vi "MI Cryostation 1.4 LV v14.vi"(6 "Temperature Set Point":dbl[unit]=4.2 min=2.0 max=350.0 step=1.0 format="%.2f", 9 "Address":string="localhost") -> (0 "Platform Stability":dbl[unit]=-0.1 format="%1.2f", 1 "Platform":dbl[unit]=-0.1 format="%1.3f", 2 "Sample Stability":dbl[unit]=-0.1 format="%1.2f", 3 "Sample":dbl[unit]=-0.1 format="%1.3f", 5 "Set Point":dbl[unit]=-0.1 format="%1.2f")   [LabVIEW 2014]
doc: "Displays data sent via TCP from Data Server.vi. Once a TCP connection is open, the VI reads 4 bytes to determine the amount of data being sent. It then reads and charts that many bytes. If an error occurs or the stop button is pressed, it sends a \"Q\" to the Data Sender to notify it to quit.\n\n<B>Note:</B> Requires the Data Server.vi located in the same library as this VI."
panel:
  out "Alarm":bool
  in  "Set Magnet Target Field":bool caption="Send"
  in  "Magnet Target Field":dbl[unit] min=-2.0 max=2.0 format="%.3f"
  in  "Magnet Disable":bool
  in  "Magnet Enable":bool
  out "Magnet Target Field":dbl[unit]=-9.999999 format="%1.3f"
  out "Magnet State":string="Unknown"
  out "Magnet":string="Magnet"
  in  "Standby":bool
  out "Heater Power":dbl[unit]=-0.1 format="%1.3f"
  out "User":dbl[unit]=-0.1 format="%1.3f"
  out "User Stability":dbl[unit]=-0.1 format="%1.2f"
  in  "Set Temperature Set Point":bool
  in  "stop":bool
  in  "Stop":bool
  in  "WarmUp":bool
  in  "CoolDown":bool
  out "Stability":string="Stability"
  out "Temperature":string="Temperature"
  out "Temperature Graph":cluster{dbl[unit], dbl[unit], dbl[unit]}(graph)
  # "Input the IP address of the Cryostation PC"
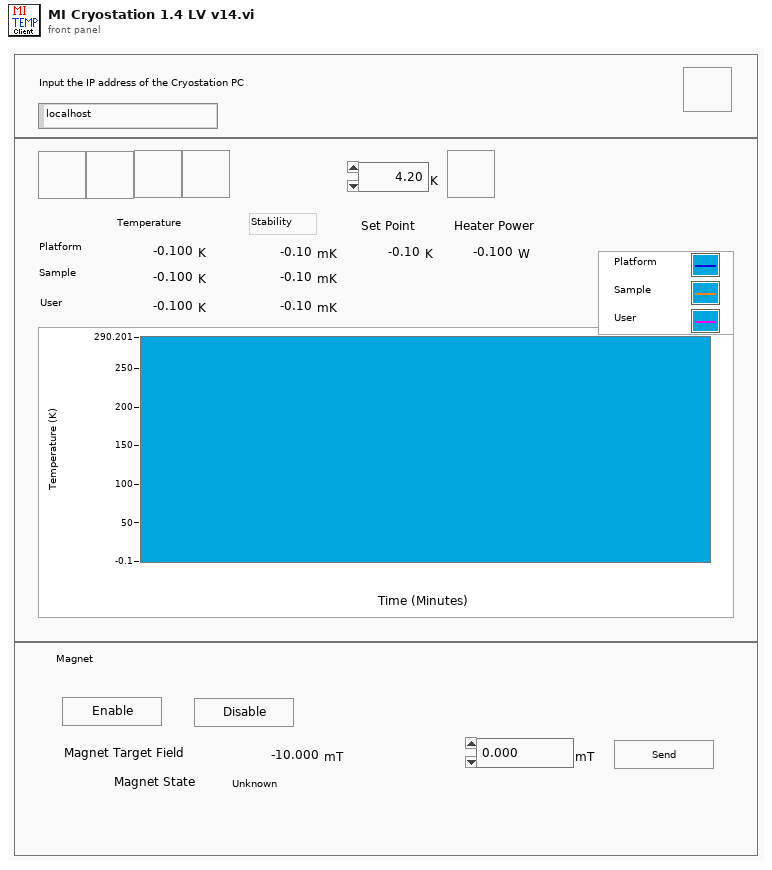
[diagram p1: front panel]
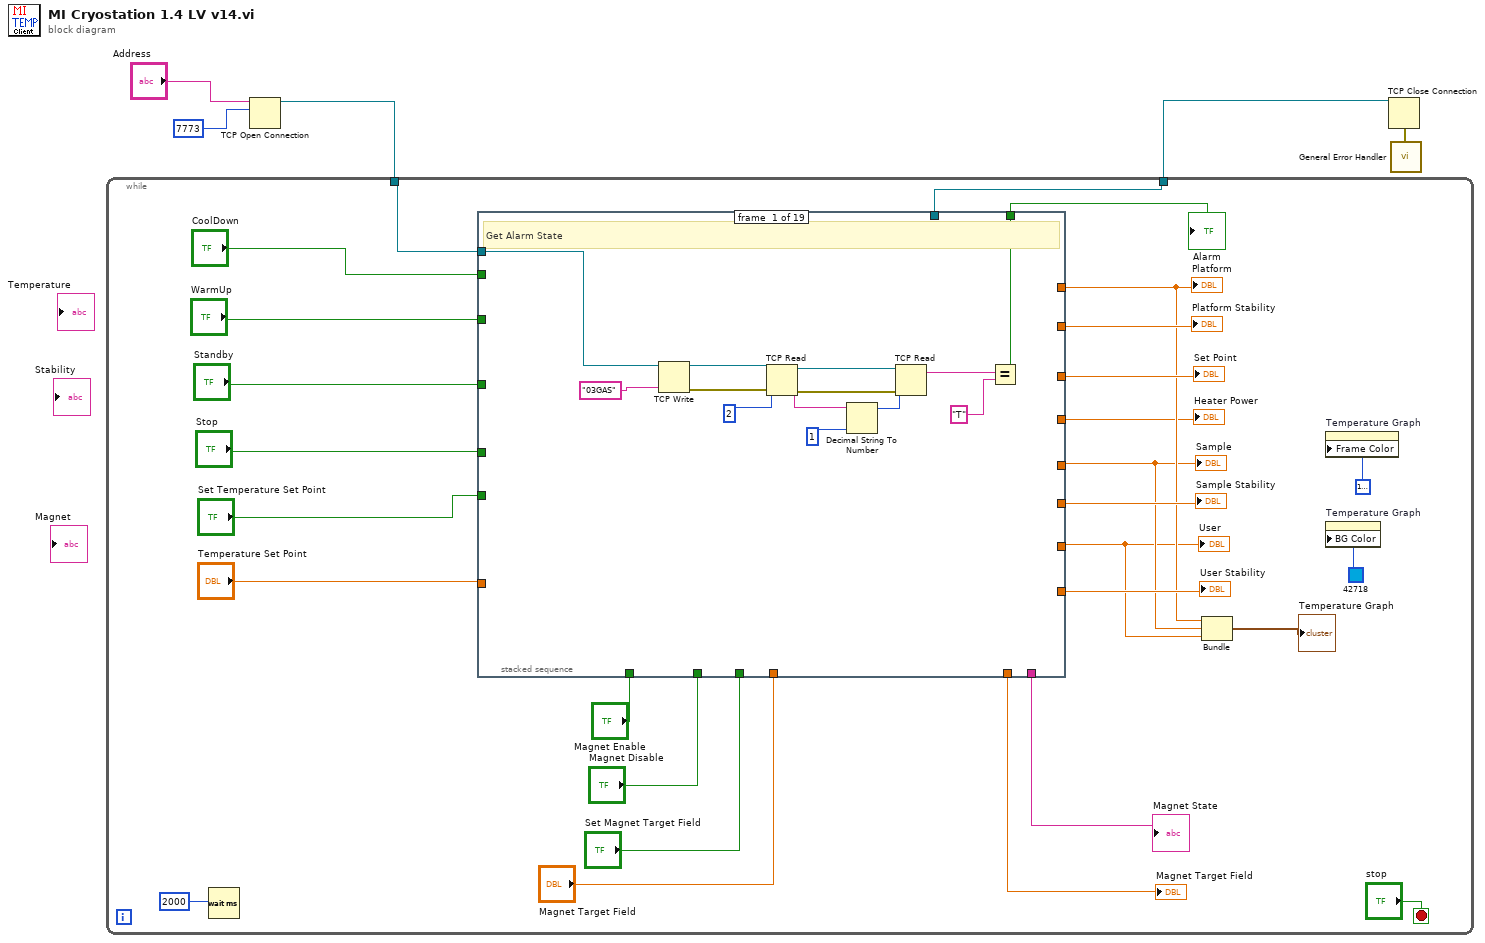
[diagram p0: block diagram]
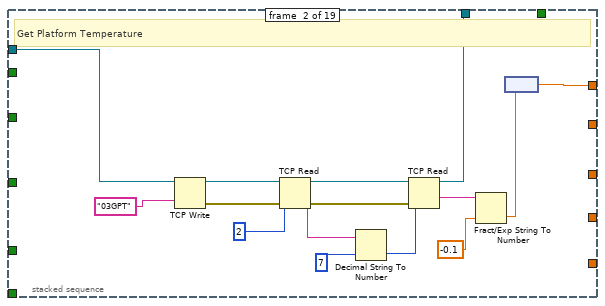
[diagram p2: hidden frame]
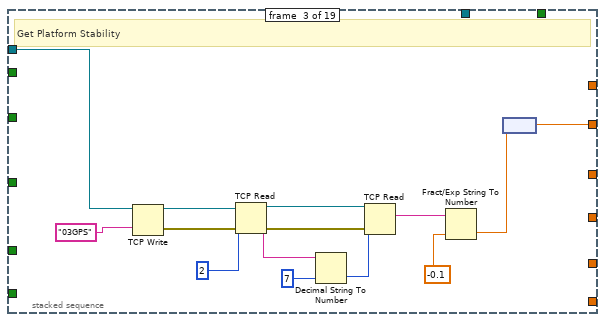
[diagram p3: hidden frame]
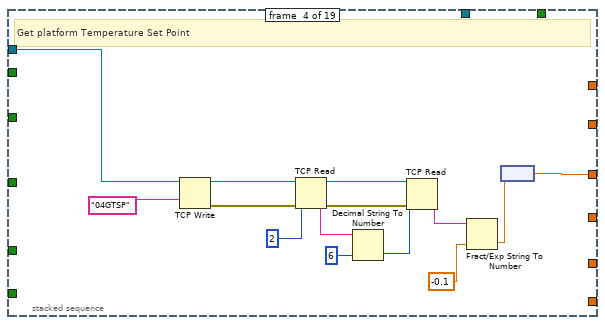
[diagram p4: hidden frame]
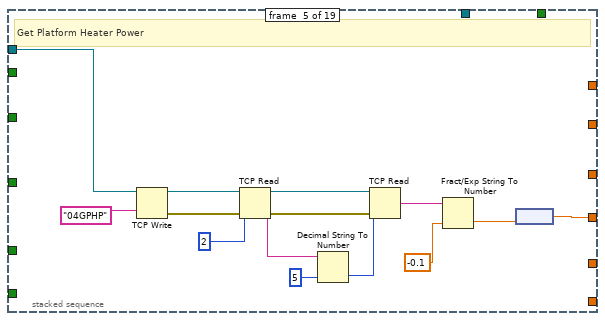
[diagram p5: hidden frame]
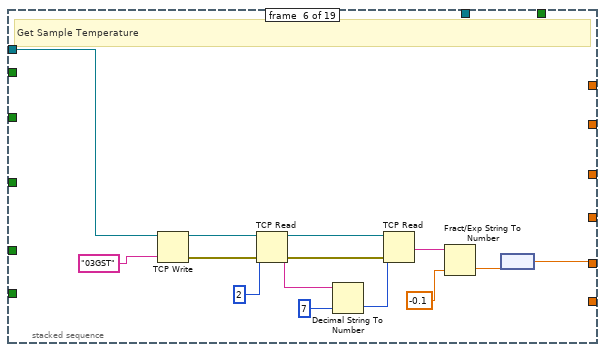
[diagram p6: hidden frame]
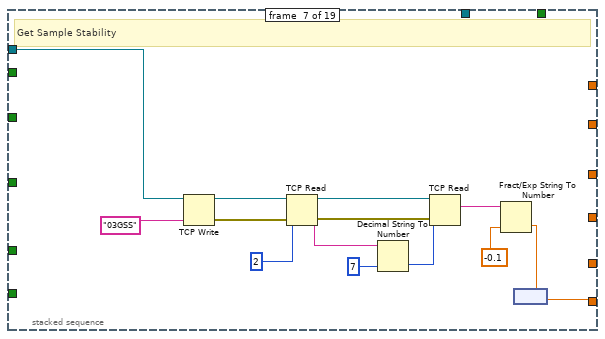
[diagram p7: hidden frame]
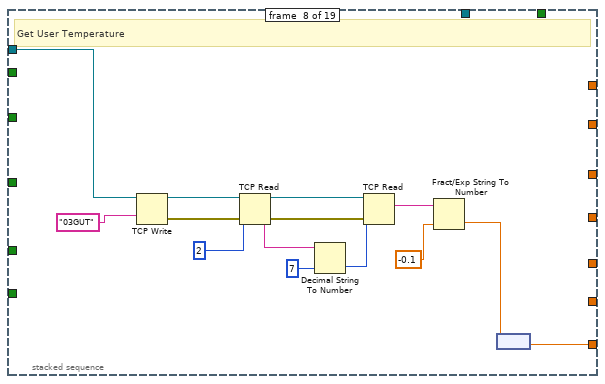
[diagram p8: hidden frame]
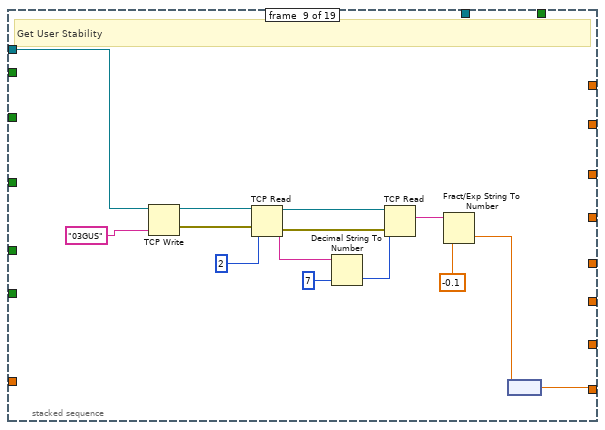
[diagram p9: hidden frame]
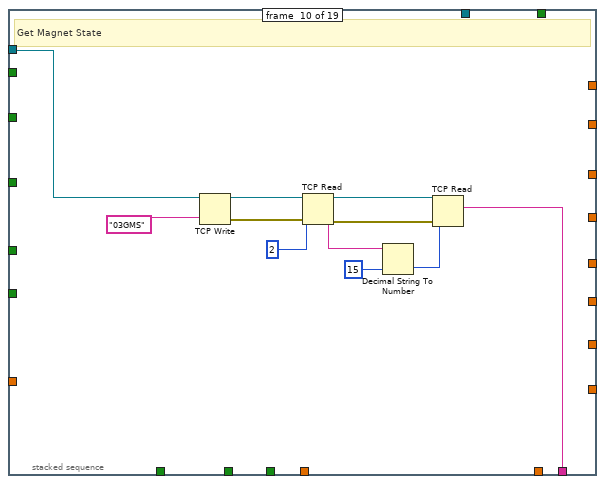
[diagram p10: hidden frame]
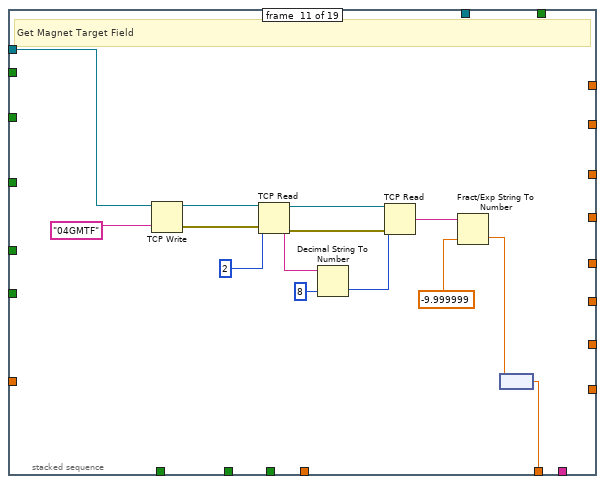
[diagram p11: hidden frame]
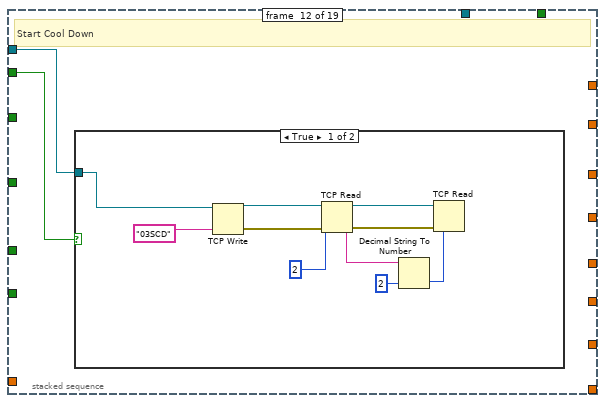
[diagram p12: hidden frame]
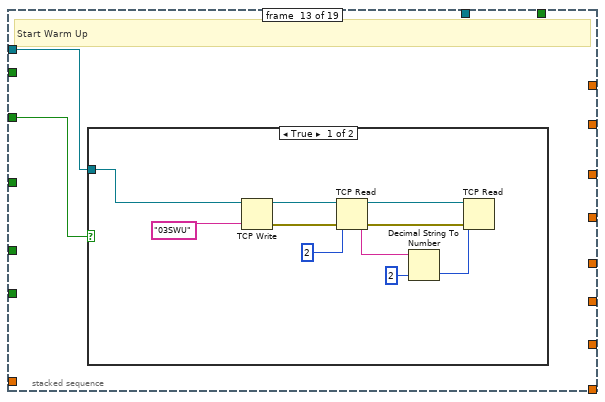
[diagram p14: hidden frame]
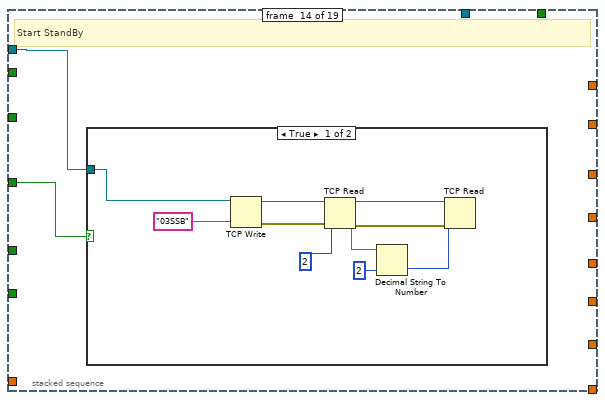
[diagram p16: hidden frame]
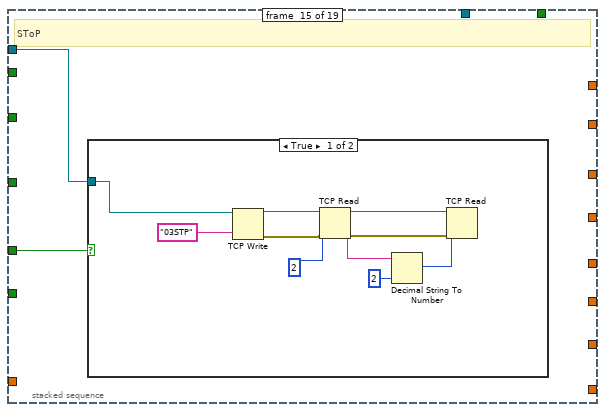
[diagram p18: hidden frame]
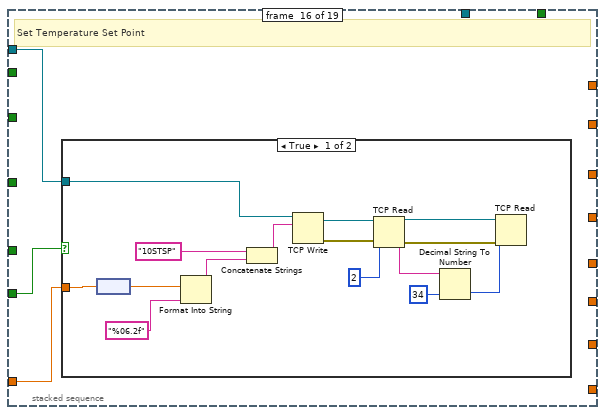
[diagram p20: hidden frame]
diagram:
  n1 = TCP Open Connection(address="Address", remote port or service name=u16 7773) -> (connection ID=w4:refnum<k5>)  [unwired: 3 in, 1 out]
  n2 = while {
    tunnel: w4 -> [w33]
    tunnel: [w30] -> w3
    stop <- "stop" stop-if-true
    n3 = Wait (ms)(milliseconds to wait=u32 2000) -> ()  [unwired: 1 out]
    n4 = stacked-sequence {
      tunnel: w33 -> [w45 w58 w72 w86 w100 w116 w128 w142 w156 w164 w177 w185 w197 w209 w221 w235 w252 w264 w277]
      tunnel: [_ _ _ w80 _ _ _ _ _ _ _ _ _ _ _ _ _ _ _] -> w26
      tunnel: "Set Temperature Set Point" -> [_ _ _ _ _ _ _ _ _ _ _ _ _ _ _ w234 _ _ _]
      tunnel: "Temperature Set Point" -> [_ _ _ _ _ _ _ _ _ _ _ _ _ _ _ w233 _ _ _]
      tunnel: [_ _ _ _ _ _ w122 _ _ _ _ _ _ _ _ _ _ _ _] -> w32
      tunnel: [_ w51 _ _ _ _ _ _ _ _ _ _ _ _ _ _ _ _ _] -> w21
      tunnel: [_ _ w67 _ _ _ _ _ _ _ _ _ _ _ _ _ _ _ _] -> w31
      tunnel: [_ _ _ _ _ w108 _ _ _ _ _ _ _ _ _ _ _ _ _] -> w20
      tunnel: [_ w53 _ _ _ _ _ _ _ _ _ _ _ _ _ _ _ _ _] -> w30
      tunnel: [_ _ _ _ _ _ _ w136 _ _ _ _ _ _ _ _ _ _ _] -> w19
      tunnel: [_ _ _ _ _ _ _ _ w150 _ _ _ _ _ _ _ _ _ _] -> w24
      tunnel: [_ _ _ _ w95 _ _ _ _ _ _ _ _ _ _ _ _ _ _] -> w6
      tunnel: "CoolDown" -> [_ _ _ _ _ _ _ _ _ _ _ w186 _ _ _ _ _ _ _]
      tunnel: "WarmUp" -> [_ _ _ _ _ _ _ _ _ _ _ _ w198 _ _ _ _ _ _]
      tunnel: "Standby" -> [_ _ _ _ _ _ _ _ _ _ _ _ _ w210 _ _ _ _ _]
      tunnel: "Stop" -> [_ _ _ _ _ _ _ _ _ _ _ _ _ _ w222 _ _ _ _]
      tunnel: [_ _ _ _ _ _ _ _ _ w163 _ _ _ _ _ _ _ _ _] -> w16
      tunnel: [_ _ _ _ _ _ _ _ _ _ w175 _ _ _ _ _ _ _ _] -> w15
      tunnel: "Magnet Enable" -> [_ _ _ _ _ _ _ _ _ _ _ _ _ _ _ _ w251 _ _]
      tunnel: "Magnet Disable" -> [_ _ _ _ _ _ _ _ _ _ _ _ _ _ _ _ _ w263 _]
      tunnel: "Set Magnet Target Field" -> [_ _ _ _ _ _ _ _ _ _ _ _ _ _ _ _ _ _ w275]
      tunnel: "Magnet Target Field" -> [_ _ _ _ _ _ _ _ _ _ _ _ _ _ _ _ _ _ w276]
      tunnel: [w40 _ _ _ _ _ _ _ _ _ _ _ _ _ _ _ _ _ _] -> w11
      frame #0 {
        # "Get Alarm State"
        n5 = TCP Write(connection ID=w45, data in="03GAS") -> (connection ID out=w39:refnum<k5>, error out=w38:errorcluster)  [unwired: 2 in, 1 out]
        n6 = TCP Read(connection ID=w39, bytes to read=2, error in (no error)=w38) -> (connection ID out=w43:refnum<k5>, data out=w34:string, error out=w37:errorcluster)  [unwired: 2 in]
        n7 = Decimal String To Number(string=w34, default (0L)=1 ("default (0 I32)")) -> (number=w35:i32)  [unwired: 1 in, 1 out]
        n8 = TCP Read(connection ID=w43, bytes to read=w35, error in (no error)=w37) -> (data out=w42:string)  [unwired: 2 in, 2 out]
        n9 = Equal?(x=w42, y="T") -> (x = y?=w40:bool)
      }
      frame #1 {
        # "Get Platform Temperature"
        n10 = TCP Write(connection ID=w58, data in="03GPT") -> (connection ID out=w61:refnum<k5>, error out=w50:errorcluster)  [unwired: 2 in, 1 out]
        n11 = TCP Read(connection ID=w61, bytes to read=2, error in (no error)=w50) -> (connection ID out=w56:refnum<k5>, data out=w57:string, error out=w49:errorcluster)  [unwired: 2 in]
        n12 = Decimal String To Number(string=w57, default (0L)=7 ("default (0 I32)")) -> (number=w55:i32)  [unwired: 1 in, 1 out]
        n13 = TCP Read(connection ID=w56, bytes to read=w55, error in (no error)=w49) -> (connection ID out=w53:refnum<k5>, data out=w54:string)  [unwired: 2 in, 1 out]
        n14 = Fract/Exp String To Number(string=w54, default (0 dbl)=-0.1 ("default (0 DBL)")) -> (number=w52:dbl)  [unwired: 2 in, 1 out]
        n15 = node(w52) -> (w51:dbl[unit])
      }
      frame #2 {
        # "Get Platform Stability"
        n16 = TCP Write(connection ID=w72, data in="03GPS") -> (connection ID out=w73:refnum<k5>, error out=w64:errorcluster)  [unwired: 2 in, 1 out]
        n17 = TCP Read(connection ID=w73, bytes to read=2, error in (no error)=w64) -> (connection ID out=w68:refnum<k5>, data out=w70:string, error out=w65:errorcluster)  [unwired: 2 in]
        n18 = Decimal String To Number(string=w70, default (0L)=7 ("default (0 I32)")) -> (number=w71:i32)  [unwired: 1 in, 1 out]
        n19 = TCP Read(connection ID=w68, bytes to read=w71, error in (no error)=w65) -> (data out=w69:string)  [unwired: 2 in, 2 out]
        n20 = Fract/Exp String To Number(string=w69, default (0 dbl)=-0.1 ("default (0 DBL)")) -> (number=w66:dbl)  [unwired: 2 in, 1 out]
        n21 = node(w66) -> (w67:dbl[unit])
      }
      frame #3 {
        # "Get platform Temperature Set Point"
        n22 = TCP Write(connection ID=w86, data in="04GTSP") -> (connection ID out=w87:refnum<k5>, error out=w79:errorcluster)  [unwired: 2 in, 1 out]
        n23 = TCP Read(connection ID=w87, bytes to read=2, error in (no error)=w79) -> (connection ID out=w84:refnum<k5>, data out=w85:string, error out=w78:errorcluster)  [unwired: 2 in]
        n24 = Decimal String To Number(string=w85, default (0L)=6 ("default (0 I32)")) -> (number=w83:i32)  [unwired: 1 in, 1 out]
        n25 = TCP Read(connection ID=w84, bytes to read=w83, error in (no error)=w78) -> (data out=w82:string)  [unwired: 2 in, 2 out]
        n26 = Fract/Exp String To Number(string=w82, default (0 dbl)=-0.1 ("default (0 DBL)")) -> (number=w81:dbl)  [unwired: 2 in, 1 out]
        n27 = node(w81) -> (w80:dbl[unit])
      }
      frame #4 {
        # "Get Platform Heater Power"
        n28 = TCP Write(connection ID=w100, data in="04GPHP") -> (connection ID out=w101:refnum<k5>, error out=w93:errorcluster)  [unwired: 2 in, 1 out]
        n29 = TCP Read(connection ID=w101, bytes to read=2, error in (no error)=w93) -> (connection ID out=w98:refnum<k5>, data out=w99:string, error out=w92:errorcluster)  [unwired: 2 in]
        n30 = Decimal String To Number(string=w99, default (0L)=5 ("default (0 I32)")) -> (number=w97:i32)  [unwired: 1 in, 1 out]
        n31 = TCP Read(connection ID=w98, bytes to read=w97, error in (no error)=w92) -> (data out=w96:string)  [unwired: 2 in, 2 out]
        n32 = Fract/Exp String To Number(string=w96, default (0 dbl)=-0.1 ("default (0 DBL)")) -> (number=w94:dbl)  [unwired: 2 in, 1 out]
        n33 = node(w94) -> (w95:dbl[unit])
      }
      frame #5 {
        # "Get Sample Temperature"
        n34 = TCP Write(connection ID=w116, data in="03GST") -> (connection ID out=w114:refnum<k5>, error out=w107:errorcluster)  [unwired: 2 in, 1 out]
        n35 = TCP Read(connection ID=w114, bytes to read=2, error in (no error)=w107) -> (connection ID out=w112:refnum<k5>, data out=w113:string, error out=w106:errorcluster)  [unwired: 2 in]
        n36 = Decimal String To Number(string=w113, default (0L)=7 ("default (0 I32)")) -> (number=w111:i32)  [unwired: 1 in, 1 out]
        n37 = TCP Read(connection ID=w112, bytes to read=w111, error in (no error)=w106) -> (data out=w110:string)  [unwired: 2 in, 2 out]
        n38 = Fract/Exp String To Number(string=w110, default (0 dbl)=-0.1 ("default (0 DBL)")) -> (number=w109:dbl)  [unwired: 2 in, 1 out]
        n39 = node(w109) -> (w108:dbl[unit])
      }
      frame #6 {
        # "Get Sample Stability"
        n40 = TCP Write(connection ID=w128, data in="03GSS") -> (connection ID out=w131:refnum<k5>, error out=w121:errorcluster)  [unwired: 2 in, 1 out]
        n41 = TCP Read(connection ID=w131, bytes to read=2, error in (no error)=w121) -> (connection ID out=w126:refnum<k5>, data out=w127:string, error out=w120:errorcluster)  [unwired: 2 in]
        n42 = Decimal String To Number(string=w127, default (0L)=7 ("default (0 I32)")) -> (number=w125:i32)  [unwired: 1 in, 1 out]
        n43 = TCP Read(connection ID=w126, bytes to read=w125, error in (no error)=w120) -> (data out=w124:string)  [unwired: 2 in, 2 out]
        n44 = Fract/Exp String To Number(string=w124, default (0 dbl)=-0.1 ("default (0 DBL)")) -> (number=w123:dbl)  [unwired: 2 in, 1 out]
        n45 = node(w123) -> (w122:dbl[unit])
      }
      frame #7 {
        # "Get User Temperature"
        n46 = TCP Write(connection ID=w142, data in="03GUT") -> (connection ID out=w145:refnum<k5>, error out=w135:errorcluster)  [unwired: 2 in, 1 out]
        n47 = TCP Read(connection ID=w145, bytes to read=2, error in (no error)=w135) -> (connection ID out=w140:refnum<k5>, data out=w141:string, error out=w134:errorcluster)  [unwired: 2 in]
        n48 = Decimal String To Number(string=w141, default (0L)=7 ("default (0 I32)")) -> (number=w139:i32)  [unwired: 1 in, 1 out]
        n49 = TCP Read(connection ID=w140, bytes to read=w139, error in (no error)=w134) -> (data out=w138:string)  [unwired: 2 in, 2 out]
        n50 = Fract/Exp String To Number(string=w138, default (0 dbl)=-0.1 ("default (0 DBL)")) -> (number=w137:dbl)  [unwired: 2 in, 1 out]
        n51 = node(w137) -> (w136:dbl[unit])
      }
      frame #8 {
        # "Get User Stability"
        n52 = TCP Write(connection ID=w156, data in="03GUS") -> (connection ID out=w159:refnum<k5>, error out=w149:errorcluster)  [unwired: 2 in, 1 out]
        n53 = TCP Read(connection ID=w159, bytes to read=2, error in (no error)=w149) -> (connection ID out=w154:refnum<k5>, data out=w155:string, error out=w148:errorcluster)  [unwired: 2 in]
        n54 = Decimal String To Number(string=w155, default (0L)=7 ("default (0 I32)")) -> (number=w153:i32)  [unwired: 1 in, 1 out]
        n55 = TCP Read(connection ID=w154, bytes to read=w153, error in (no error)=w148) -> (data out=w152:string)  [unwired: 2 in, 2 out]
        n56 = Fract/Exp String To Number(string=w152, default (0 dbl)=-0.1 ("default (0 DBL)")) -> (number=w151:dbl)  [unwired: 2 in, 1 out]
        n57 = node(w151) -> (w150:dbl[unit])
      }
      frame #9 {
        # "Get Magnet State"
        n58 = TCP Write(connection ID=w164, data in="03GMS") -> (connection ID out=w170:refnum<k5>, error out=w162:errorcluster)  [unwired: 2 in, 1 out]
        n59 = TCP Read(connection ID=w170, bytes to read=2, error in (no error)=w162) -> (connection ID out=w166:refnum<k5>, data out=w167:string, error out=w161:errorcluster)  [unwired: 2 in]
        n60 = Decimal String To Number(string=w167, default (0L)=15 ("default (0 I32)")) -> (number=w165:i32)  [unwired: 1 in, 1 out]
        n61 = TCP Read(connection ID=w166, bytes to read=w165, error in (no error)=w161) -> (data out=w163:string)  [unwired: 2 in, 2 out]
      }
      frame #10 {
        # "Get Magnet Target Field"
        n62 = TCP Write(connection ID=w177, data in="04GMTF") -> (connection ID out=w179:refnum<k5>, error out=w174:errorcluster)  [unwired: 2 in, 1 out]
        n63 = TCP Read(connection ID=w179, bytes to read=2, error in (no error)=w174) -> (connection ID out=w183:refnum<k5>, data out=w182:string, error out=w173:errorcluster)  [unwired: 2 in]
        n64 = Decimal String To Number(string=w182, default (0L)=8 ("default (0 I32)")) -> (number=w184:i32)  [unwired: 1 in, 1 out]
        n65 = TCP Read(connection ID=w183, bytes to read=w184, error in (no error)=w173) -> (data out=w178:string)  [unwired: 2 in, 2 out]
        n66 = Fract/Exp String To Number(string=w178, default (0 dbl)=-9.999999 ("default (0 DBL)")) -> (number=w176:dbl)  [unwired: 2 in, 1 out]
        n67 = node(w176) -> (w175:dbl[unit])
      }
      frame #11 {
        # "Start Cool Down"
        n68 = case shown="True" w186 {
          tunnel: w185 -> [w196 _]
          frame True {
            n69 = TCP Write(connection ID=w196, data in="03SCD") -> (connection ID out=w195:refnum<k5>, error out=w189:errorcluster)  [unwired: 2 in, 1 out]
            n70 = TCP Read(connection ID=w195, bytes to read=2 ("timeout ms (25000)"), error in (no error)=w189) -> (connection ID out=w190:refnum<k5>, data out=w192:string, error out=w188:errorcluster)  [unwired: 2 in]
            n71 = Decimal String To Number(string=w192, default (0L)=2 ("default (0 I32)")) -> (number=w191:i32)  [unwired: 1 in, 1 out]
            n72 = TCP Read(connection ID=w190, bytes to read=w191, error in (no error)=w188) -> ()  [unwired: 2 in, 3 out]
          }
          frame False {
          }
        }
      }
      frame #12 {
        # "Start Warm Up"
        n73 = case shown="True" w198 {
          tunnel: w197 -> [w208 _]
          frame True {
            n74 = TCP Write(connection ID=w208, data in="03SWU") -> (connection ID out=w207:refnum<k5>, error out=w201:errorcluster)  [unwired: 2 in, 1 out]
            n75 = TCP Read(connection ID=w207, bytes to read=2 ("timeout ms (25000)"), error in (no error)=w201) -> (connection ID out=w203:refnum<k5>, data out=w202:string, error out=w200:errorcluster)  [unwired: 2 in]
            n76 = Decimal String To Number(string=w202, default (0L)=2 ("default (0 I32)")) -> (number=w204:i32)  [unwired: 1 in, 1 out]
            n77 = TCP Read(connection ID=w203, bytes to read=w204, error in (no error)=w200) -> ()  [unwired: 2 in, 3 out]
          }
          frame False {
          }
        }
      }
      frame #13 {
        # "Start StandBy"
        n78 = case shown="True" w210 {
          tunnel: w209 -> [w220 _]
          frame True {
            n79 = TCP Write(connection ID=w220, data in="03SSB") -> (connection ID out=w219:refnum<k5>, error out=w213:errorcluster)  [unwired: 2 in, 1 out]
            n80 = TCP Read(connection ID=w219, bytes to read=2 ("timeout ms (25000)"), error in (no error)=w213) -> (connection ID out=w214:refnum<k5>, data out=w215:string, error out=w212:errorcluster)  [unwired: 2 in]
            n81 = Decimal String To Number(string=w215, default (0L)=2 ("default (0 I32)")) -> (number=w216:i32)  [unwired: 1 in, 1 out]
            n82 = TCP Read(connection ID=w214, bytes to read=w216, error in (no error)=w212) -> ()  [unwired: 2 in, 3 out]
          }
          frame False {
          }
        }
      }
      frame #14 {
        # "SToP"
        n83 = case shown="True" w222 {
          tunnel: w221 -> [w232 _]
          frame True {
            n84 = TCP Write(connection ID=w232, data in="03STP") -> (connection ID out=w231:refnum<k5>, error out=w225:errorcluster)  [unwired: 2 in, 1 out]
            n85 = TCP Read(connection ID=w231, bytes to read=2 ("timeout ms (25000)"), error in (no error)=w225) -> (connection ID out=w226:refnum<k5>, data out=w227:string, error out=w224:errorcluster)  [unwired: 2 in]
            n86 = Decimal String To Number(string=w227, default (0L)=2 ("default (0 I32)")) -> (number=w228:i32)  [unwired: 1 in, 1 out]
            n87 = TCP Read(connection ID=w226, bytes to read=w228, error in (no error)=w224) -> ()  [unwired: 2 in, 3 out]
          }
          frame False {
          }
        }
      }
      frame #15 {
        # "Set Temperature Set Point"
        n88 = case shown="True" w234 {
          tunnel: w233 -> [w240 _]
          tunnel: w235 -> [w246 _]
          frame True {
            n89 = node(w240) -> (w239:dbl)
            n90 = Format Into String(format string="%06.2f", w239) -> (resulting string=w248:string)  [unwired: 2 in, 1 out]
            n91 = Concatenate Strings("10STSP", w248) -> (w247:string)
            n92 = TCP Write(connection ID=w246, data in=w247) -> (connection ID out=w245:refnum<k5>, error out=w238:errorcluster)  [unwired: 2 in, 1 out]
            n93 = TCP Read(connection ID=w245, bytes to read=2 ("timeout ms (25000)"), error in (no error)=w238) -> (connection ID out=w243:refnum<k5>, data out=w242:string, error out=w237:errorcluster)  [unwired: 2 in]
            n94 = Decimal String To Number(string=w242, default (0L)=34 ("default (0 I32)")) -> (number=w241:i32)  [unwired: 1 in, 1 out]
            n95 = TCP Read(connection ID=w243, bytes to read=w241, error in (no error)=w237) -> ()  [unwired: 2 in, 3 out]
          }
          frame False {
          }
        }
      }
      frame #16 {
        # "Set Magnet Enabled"
        n96 = case shown="True" w251 {
          tunnel: w252 -> [w262 _]
          frame True {
            n97 = TCP Write(connection ID=w262, data in="03SME") -> (connection ID out=w261:refnum<k5>, error out=w255:errorcluster)  [unwired: 2 in, 1 out]
            n98 = TCP Read(connection ID=w261, bytes to read=2 ("timeout ms (25000)"), error in (no error)=w255) -> (connection ID out=w256:refnum<k5>, data out=w257:string, error out=w254:errorcluster)  [unwired: 2 in]
            n99 = Decimal String To Number(string=w257, default (0L)=18 ("default (0 I32)")) -> (number=w258:i32)  [unwired: 1 in, 1 out]
            n100 = TCP Read(connection ID=w256, bytes to read=w258, error in (no error)=w254) -> ()  [unwired: 2 in, 3 out]
          }
          frame False {
          }
        }
      }
      frame #17 {
        # "Set Magnet Disabled"
        n101 = case shown="True" w263 {
          tunnel: w264 -> [w274 _]
          frame True {
            n102 = TCP Write(connection ID=w274, data in="03SMD") -> (connection ID out=w273:refnum<k5>, error out=w267:errorcluster)  [unwired: 2 in, 1 out]
            n103 = TCP Read(connection ID=w273, bytes to read=2 ("timeout ms (25000)"), error in (no error)=w267) -> (connection ID out=w268:refnum<k5>, data out=w269:string, error out=w266:errorcluster)  [unwired: 2 in]
            n104 = Decimal String To Number(string=w269, default (0L)=19 ("default (0 I32)")) -> (number=w270:i32)  [unwired: 1 in, 1 out]
            n105 = TCP Read(connection ID=w268, bytes to read=w270, error in (no error)=w266) -> ()  [unwired: 2 in, 3 out]
          }
          frame False {
          }
        }
      }
      frame #18 {
        # "Set Magnet Target Field"
        n106 = case shown="True" w275 {
          tunnel: w276 -> [w282 _]
          tunnel: w277 -> [w288 _]
          frame True {
            n107 = node(w282) -> (w281:dbl)
            n108 = Format Into String(format string="%+08.6f", w281) -> (resulting string=w290:string)  [unwired: 2 in, 1 out]
            n109 = Concatenate Strings("13SMTF", w290) -> (w289:string)
            n110 = TCP Write(connection ID=w288, data in=w289) -> (connection ID out=w287:refnum<k5>, error out=w280:errorcluster)  [unwired: 2 in, 1 out]
            n111 = TCP Read(connection ID=w287, bytes to read=2 ("timeout ms (25000)"), error in (no error)=w280) -> (connection ID out=w285:refnum<k5>, data out=w284:string, error out=w279:errorcluster)  [unwired: 2 in]
            n112 = Decimal String To Number(string=w284, default (0L)=34 ("default (0 I32)")) -> (number=w283:i32)  [unwired: 1 in, 1 out]
            n113 = TCP Read(connection ID=w285, bytes to read=w283, error in (no error)=w279) -> ()  [unwired: 2 in, 3 out]
          }
          frame False {
          }
        }
      }
    }
    "Set Point" <- w26
    "Sample Stability" <- w32
    "Platform" <- w21
    "Platform Stability" <- w31
    "Sample" <- w20
    "Heater Power" <- w6
    "User Stability" <- w24
    "User" <- w19
    "Magnet State" <- w16
    "Magnet Target Field" <- w15
    "Alarm" <- w11
    n114 = Bundle(w21, w20, w19) -> (→"Temperature Graph":cluster{dbl[unit], dbl[unit], dbl[unit]})  [unwired: 1 in]
    n115 = property on="Temperature Graph" class="WFChart (strict)"("Frame Color"=u32 16777226) -> ()  [unwired: 2 in, 2 out]
    n116 = property on="Temperature Graph" class="WFChart (strict)"("BG Color"=u32 42718 ("Color Box")) -> ()  [unwired: 2 in, 2 out]
  }
  n117 = TCP Close Connection(connection ID=w3) -> (error out=w2:errorcluster)  [unwired: 2 in, 1 out]
  n118 = call <vilib>:"General Error Handler.vi"("error in (no error)"=w2) -> ()  [unwired: 2 in, 13 out]
